vi "Square.vi"(11 "Min/Max Voltage":dbl format="%#_13g") -> (0 "Rate":dbl=200000.0, 2 "Waveform Graph":dbl[][](graph), 3 "XY Graph":cluster{"Y":dbl[], "X":dbl[]}(graph))   [LabVIEW 2021]
doc: "This VI enables to display the Square optotype.\n\nInput:\n(1) Min/Max Voltage - the absolute value of the Voltage. Due to this parameter, the size of the optotype can be changed. Voltage about 10V is not allowed.\n\nOutputs: \n(1) XY Graph - the optotype data, to display the pattern.\n(2) Scanners trajectories - the XY data for the Scanners.\n(3) Rate - the rate parameter equal to 200000."
uses:
  <vilib>/Analysis/1siggen.llb/Ramp Pattern by Samples.vi
  <vilib>/Analysis/NI_AALBase.lvlib
panel:
  in  "Number of samples":i32=100
  in  "Number of lines":i32=50
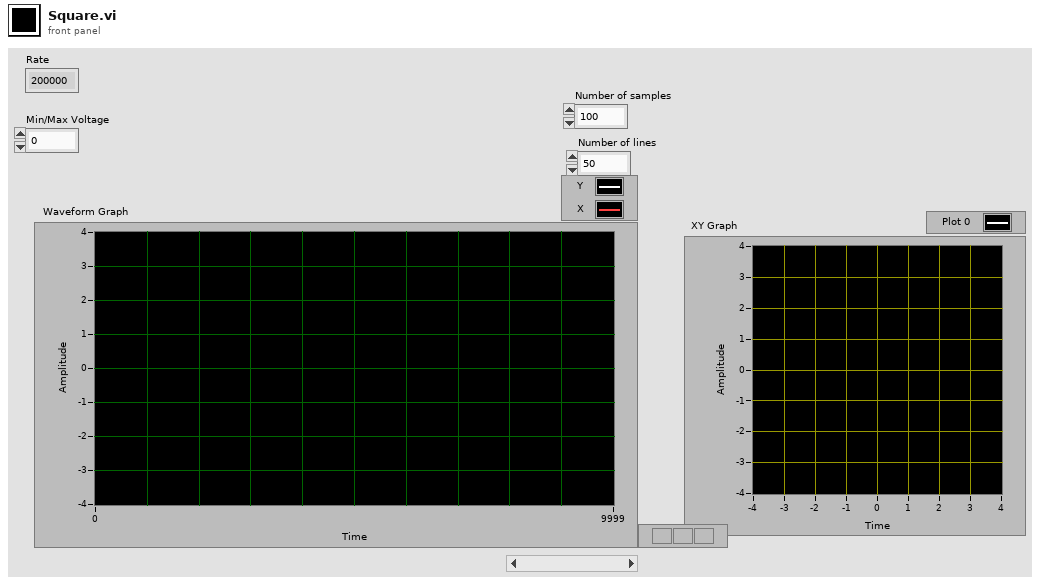
[diagram p1: front panel]
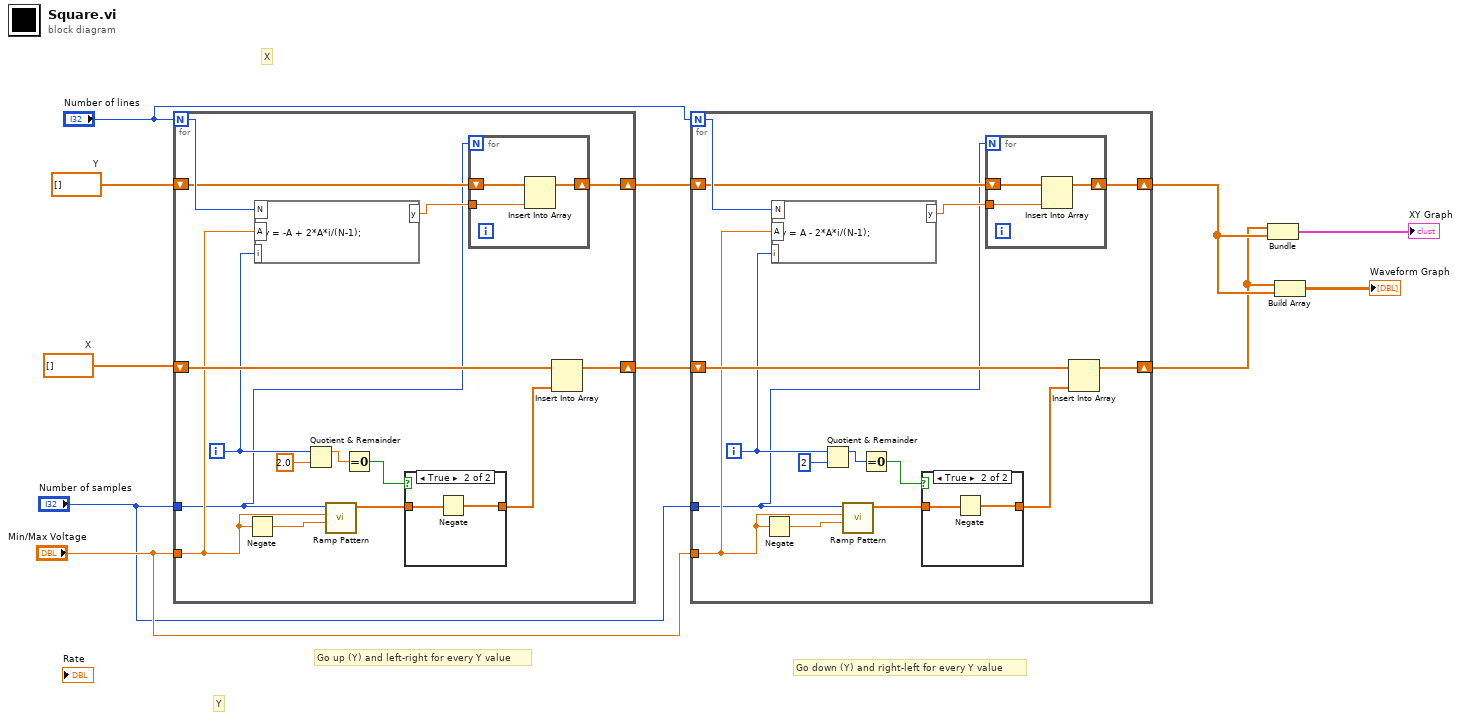
[diagram p0: block diagram]
diagram:
  w11 = dbl[] []  # X
  w10 = dbl[] []  # Y
  # "Go down (Y) and right-left for every Y value"
  # "Go up (Y) and left-right for every Y value"
  # "Y"
  # "X"
  n1 = for {
    N: "Number of lines" -> [w22]
    tunnel: "Number of samples" -> [w13]
    tunnel: "Min/Max Voltage" -> [w16]
    shift-right: [w19] -> w6
    shift-left: w11 -> [w20]
    shift-right: [w17] -> w7
    shift-left: w10 -> [w18]
    i -> [w14]
    n2 = Negate(x=w16) -> (-x=w26:dbl)
    n3 = formula code="y = -A + 2*A*i/(N-1);"("A"=w16, "i"=w14, "N"=w22) -> ("y"=w15:dbl)
    n4 = Quotient & Remainder(x=w14, y=2.0) -> (x-y*floor(x/y)=w12:dbl)  [unwired: 1 out]
    n5 = call-poly <vilib>:"Ramp Pattern.vi"("start"=w26, "end"=w16, "samples"=w13) -> ("Ramp Pattern"=w25:dbl[])  [unwired: 7 in, 1 out]
    n6 = Equal To 0?(x=w12) -> (x = 0?=w23:bool)
    n7 = case shown="True" w23 {
      tunnel: w25 -> [w30 w32]
      tunnel: [w30 w31] -> w21
      frame False {
      }
      frame True {
        n8 = Negate(x=w32) -> (-x=w31:dbl[])
      }
    }
    n9 = for {
      N: w13 -> [_]
      tunnel: w15 -> [w28]
      shift-right: [w29] -> w17
      shift-left: w18 -> [w27]
      n10 = Insert Into Array(array=w27, new element=w28) -> (w29:dbl[])  [unwired: 1 in]
    }
    n11 = Insert Into Array(array=w20, new element=w21) -> (w19:dbl[])  [unwired: 1 in]
  }
  n12 = for {
    N: "Number of lines" -> [w43]
    tunnel: "Number of samples" -> [w34]
    tunnel: "Min/Max Voltage" -> [w37]
    shift-right: [w40] -> w2
    shift-left: w6 -> [w41]
    shift-right: [w38] -> w3
    shift-left: w7 -> [w39]
    i -> [w35]
    n13 = Negate(x=w37) -> (-x=w47:dbl)
    n14 = formula code="y = A - 2*A*i/(N-1);"("A"=w37, "i"=w35, "N"=w43) -> ("y"=w36:dbl)
    n15 = Quotient & Remainder(x=w35, y=2) -> (x-y*floor(x/y)=w33:i32)  [unwired: 1 out]
    n16 = call-poly <vilib>:"Ramp Pattern.vi"("start"=w47, "end"=w37, "samples"=w34) -> ("Ramp Pattern"=w46:dbl[])  [unwired: 7 in, 1 out]
    n17 = Equal To 0?(x=w33) -> (x = 0?=w44:bool)
    n18 = case shown="True" w44 {
      tunnel: w46 -> [w51 w53]
      tunnel: [w51 w52] -> w42
      frame False {
      }
      frame True {
        n19 = Negate(x=w53) -> (-x=w52:dbl[])
      }
    }
    n20 = for {
      N: w34 -> [_]
      tunnel: w36 -> [w49]
      shift-right: [w50] -> w38
      shift-left: w39 -> [w48]
      n21 = Insert Into Array(array=w48, new element=w49) -> (w50:dbl[])  [unwired: 1 in]
    }
    n22 = Insert Into Array(array=w41, new element=w42) -> (w40:dbl[])  [unwired: 1 in]
  }
  n23 = Bundle("X"=w2, "Y"=w3) -> (→"XY Graph":cluster{"X":dbl[], "Y":dbl[]})  [unwired: 1 in]
  n24 = Build Array(w2, w3) -> (→"Waveform Graph":dbl[][])
